vi "OpenConvert Examples.vi"() -> ()   [LabVIEW 2013]
uses:
  source/Conversions/OpenConvert.lvlib
panel:
  out "Original Dimensions":u32[](array[numeric])
  out "Array Elements":variant[](array[variant])
  out "Relative Path":bool
  out "Absolute Path":bool
  out "Not A Path":bool
  out "Cluster Elements":variant[](array[variant])
  out "rebuilt relative path string":string
  out "rebuilt absolute path":path
  out "rebuilt relative path":path
  out "relatiive path":path
  out "absolute path":path
  out "relative path string":string
  out "absolute path string":string
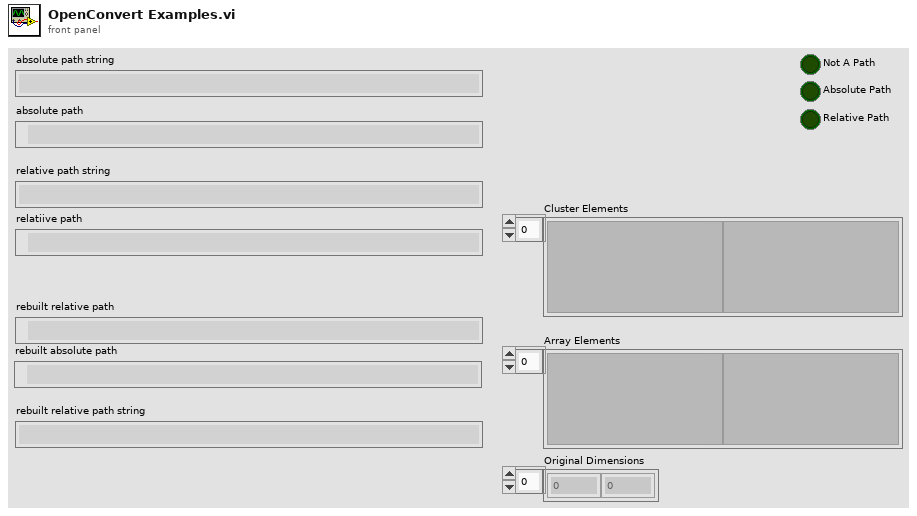
[diagram p1: front panel]
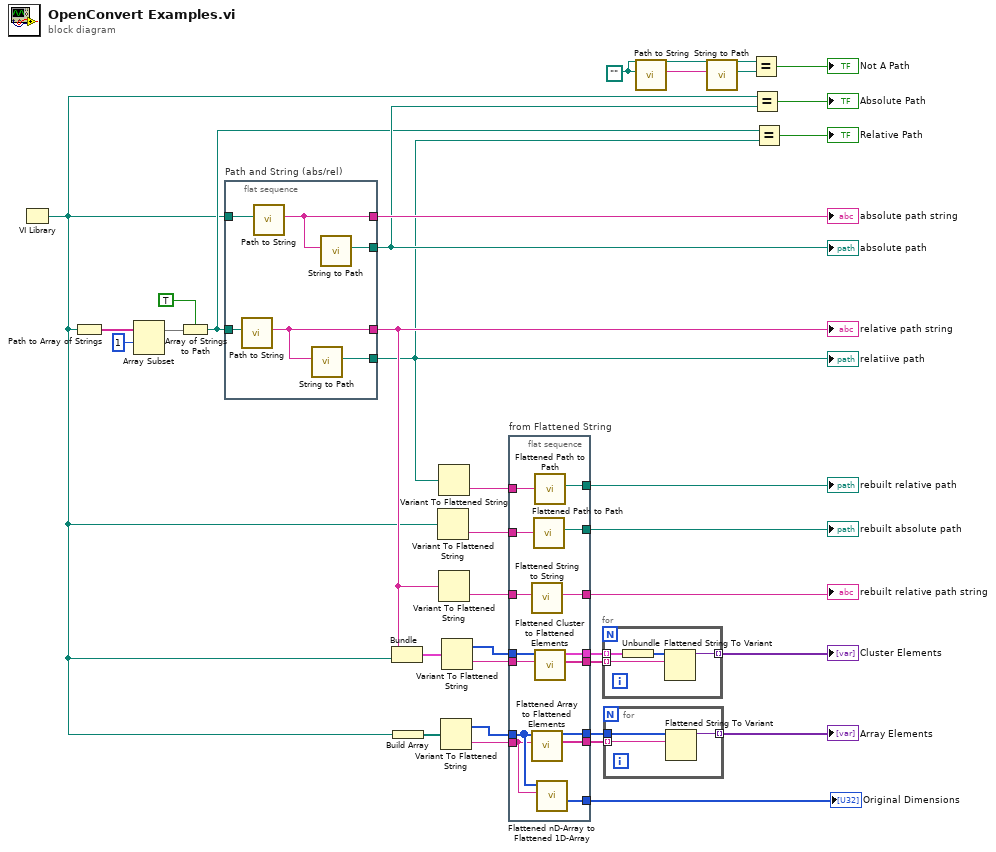
[diagram p0: block diagram]
diagram:
  w15 = path ""
  n1 = VI Library() -> (path=w8:path)
  n2 = Path to Array of Strings(0:w8) -> (2:w35:string[])  [unwired: 1 out]
  n3 = Array Subset(array=w35, index=1) -> (w34:string[])  [unwired: 1 in]
  n4 = Array of Strings to Path(0:w34, 1:TRUE ("relative")) -> (2:w10:path)
  n5 = flat-sequence "Path and String (abs/rel)" {
    tunnel: w10 -> [w41]
    tunnel: [w40] -> w31
    tunnel: [w39] -> w13
    tunnel: [w38] -> w9
    tunnel: w8 -> [w37]
    tunnel: [w36] -> w18
    frame #0 {
      n6 = call "Path to String.vi"("specific path"=w41) -> ("common path"=w36:string)  [unwired: 10 in]
      n7 = call "Path to String.vi"("specific path"=w37) -> ("common path"=w40:string)  [unwired: 10 in]
      n8 = call "String to Path.vi"("common path"=w36) -> ("specific path"=w38:path)  [unwired: 10 in]
      n9 = call "String to Path.vi"("common path"=w40) -> ("specific path"=w39:path)  [unwired: 10 in]
    }
  }
  n10 = Bundle("common path"=w18, "path"=w8) -> (w24:cluster{"common path":string, "path":path})  [unwired: 1 in]
  n11 = Build Array(w8) -> (w7:path[])
  n12 = Variant To Flattened String(Variant=w8) -> (data string=w27:string)  [unwired: 1 out]
  n13 = Variant To Flattened String(Variant=w9) -> (data string=w30:string)  [unwired: 1 out]
  n14 = Variant To Flattened String(Variant=w18) -> (data string=w26:string)  [unwired: 1 out]
  n15 = Variant To Flattened String(Variant=w7) -> (data string=w5:string, 1:w6:i16[])
  n16 = Variant To Flattened String(Variant=w24) -> (data string=w22:string, 1:w23:i16[])
  n17 = flat-sequence "from Flattened String" {
    tunnel: w30 -> [w56]
    tunnel: [w55] -> w29
    tunnel: [w54] -> w28
    tunnel: w27 -> [w53]
    tunnel: w26 -> [w52]
    tunnel: [w51] -> w25
    tunnel: w23 -> [w50]
    tunnel: w22 -> [w49]
    tunnel: [w48] -> w21
    tunnel: [w47] -> w20
    tunnel: w6 -> [w44]
    tunnel: w5 -> [w43]
    tunnel: [w46] -> w4
    tunnel: [w45] -> w3
    tunnel: [w42] -> w1
    frame #0 {
      n18 = call "Flattened String to String.vi"("Flattened String"=w52) -> ("String"=w51:string)  [unwired: 9 in, 1 out]
      n19 = call "Flattened Array to Flattened Elements.vi"("Flattened Array String"=w43, "Array Type Descriptor"=w44) -> ("Flattened Array Elements"=w45:string[], "Array Element Type Descriptor"=w46:i16[])  [unwired: 8 in]
      n20 = call "Flattened Path to Path.vi"("Flattened Path String"=w53) -> ("path"=w54:path)  [unwired: 10 in]
      n21 = call "Flattened Path to Path.vi"("Flattened Path String"=w56) -> ("path"=w55:path)  [unwired: 10 in]
      n22 = call "Flattened Cluster to Flattened Elements.vi"("Flattened Cluster"=w49, "Cluster Type Descriptor"=w50) -> ("Flattened Cluster Elements"=w47:string[], "Elements Type Descriptor"=w48:cluster{"Type Descriptor":i16[]}[])  [unwired: 8 in]
      n23 = call "Flattened nD-Array to Flattened 1D-Array.vi"("Flattened nD Array"=w43, "nD Array Type Descriptor"=w44) -> ("Original Dimensions"=w42:u32[])  [unwired: 7 in, 2 out]
    }
  }
  n24 = for {
    tunnel: w21 -> [w59] mode=indexing
    tunnel: w20 -> [w60] mode=indexing
    tunnel: [w57] -> w19 mode=indexing
    n25 = Unbundle(w59) -> ("Type Descriptor"=w58:i16[])
    n26 = Flattened String To Variant(6:w60, 7:w58) -> (3:w57:variant)  [unwired: 1 in, 1 out]
  }
  "Cluster Elements" <- w19
  n27 = for {
    tunnel: w4 -> [w61]
    tunnel: w3 -> [w63] mode=indexing
    tunnel: [w62] -> w2 mode=indexing
    n28 = Flattened String To Variant(6:w63, 7:w61) -> (3:w62:variant)  [unwired: 1 in, 1 out]
  }
  "Array Elements" <- w2
  n29 = call "Path to String.vi"("specific path"=w15) -> ("common path"=w17:string)  [unwired: 10 in]
  n30 = call "String to Path.vi"("common path"=w17) -> ("specific path"=w16:path)  [unwired: 10 in]
  n31 = Equal?(x=w15, y=w16) -> (x = y?=→"Not A Path":bool)
  n32 = Equal?(x=w8, y=w13) -> (x = y?=→"Absolute Path":bool)
  n33 = Equal?(x=w10, y=w9) -> (x = y?=→"Relative Path":bool)
  "absolute path string" <- w31
  "relative path string" <- w18
  "absolute path" <- w13
  "relatiive path" <- w9
  "rebuilt relative path" <- w29
  "rebuilt absolute path" <- w28
  "rebuilt relative path string" <- w25
  "Original Dimensions" <- w1
